vi "EdgeCounter.vi"(1 "DetectorType":T1, 2 "Reset":bool, 4 "Input":bool) -> (0 "EdgeCount":u32)   [LabVIEW 2018]
uses:
  TypeDefs/EdgeDetector_Type.ctl
  ArgosLib.lvlib
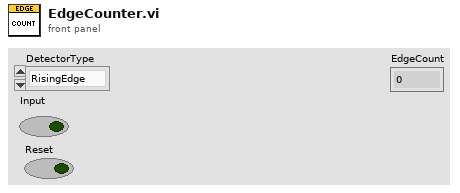
[diagram p1: front panel]
types:
  T1 = typedef "ArgosLib.lvlib/EdgeDetector_Type.ctl" = enum16{"RisingEdge", "FallingEdge", "Both"}
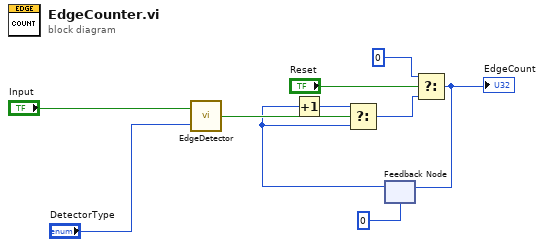
[diagram p0: block diagram]
diagram:
  n1 = call "EdgeDetector.vi"("DetectorType"="DetectorType", "Input"="Input") -> ("Edge"=w8:bool)
  n2 = feedback #1(u32 0) -> (w4:u32)
  n3 = Increment(x=w4) -> (x+1=w3:u32)
  n4 = Select(t=w3, s=w8, f=w4) -> (s? t:f=w2:u32)
  n5 = Select(t=u32 0, s="Reset", f=w2) -> (s? t:f=w5:u32)
  "EdgeCount" <- w5
  n6 = feedback-in #1(w5) -> ()
